vi "encodeFloat.vi"(8 "error in (no error)":errorcluster, 10 "Variant":variant) -> (0 "error out":errorcluster, 2 "Array":u8[](array[numeric]) format="%.0x")   [LabVIEW 2016, in "MsgPack.lvlib"]
uses:
  MsgPack.lvlib
  <vilib>/Utility/Data Type/NI_Data Type.lvlib
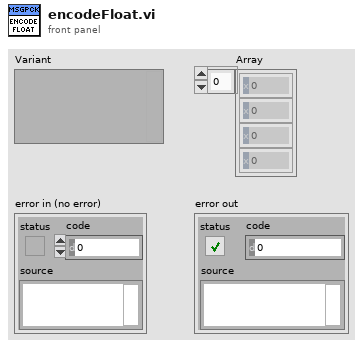
[diagram p1: front panel]
types:
  T1 = typedef "NI_Data Type.lvlib/Data Type.ctl" = enum8{"Invalid Type", "Void", "I8", "I16", "I32", "I64", "U8", "U16", "U32", "U64", "Single Float", "Double Float", "Extended Float", "Single Complex", "Double Complex", "Extended Complex", "Enum U8", "Enum U16", "Enum U32", "Enum U64", "Single Float With Unit", "Double Float With Unit", "Extended Float With Unit", "Single Complex with Unit", "Double Complex with Unit", "Extended Complex with Unit", "Boolean", "String", "Path", "Picture", "Tag", "Array", "Cluster", "Variant", "LV Variant", "Waveform", "Timestamp", "Digital Waveform", "Digital Data", "ExpressData", "Refnum", "External Data", "VI", "Poly VI", "LabVIEW Class Instance", "Fixed Point"}
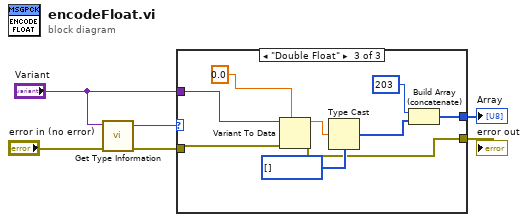
[diagram p0: block diagram]
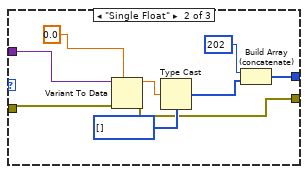
[diagram p3: hidden frame]
diagram:
  n1 = call <vilib>:"Get Type Information.vi"("error in (no error)"="error in (no error)", "Variant"="Variant") -> ("error out"=w5:errorcluster, "Type"=w6:T1)  [unwired: 5 in, 3 out]
  n2 = case shown="\"Double Float\"" w6 {
    tunnel: w5 -> [w7 w16 w25]
    tunnel: "Variant" -> [_ w15 w24]
    tunnel: [_ w10 w19] -> w3
    tunnel: [w7 w9 w18] -> w2
    frame "Invalid Type", Default {
    }
    frame "Single Float" {
      n3 = Variant To Data(error in=w16, type=sgl 0.0, Variant=w15) -> (data=w13:sgl, error out=w9:errorcluster)
      n4 = Type Cast(type=u8[] [], x=w13) -> (*(type *) &x=w11:u8[])
      n5 = Build Array (concatenate)(u8 202, w11) -> (w10:u8[])
    }
    frame "Double Float" {
      n6 = Variant To Data(error in=w25, type=0.0, Variant=w24) -> (data=w22:dbl, error out=w18:errorcluster)
      n7 = Type Cast(type=u8[] [], x=w22) -> (*(type *) &x=w20:u8[])
      n8 = Build Array (concatenate)(u8 203, w20) -> (w19:u8[])
    }
  }
  "Array" <- w3
  "error out" <- w2
